vi "Part 1.vi"(7 "Steps":i32=10, 11 "Input":string) -> (3 "Output":i64)   [LabVIEW 2021]
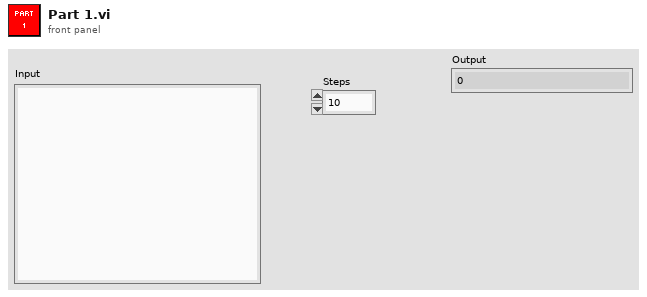
[diagram p1: front panel]
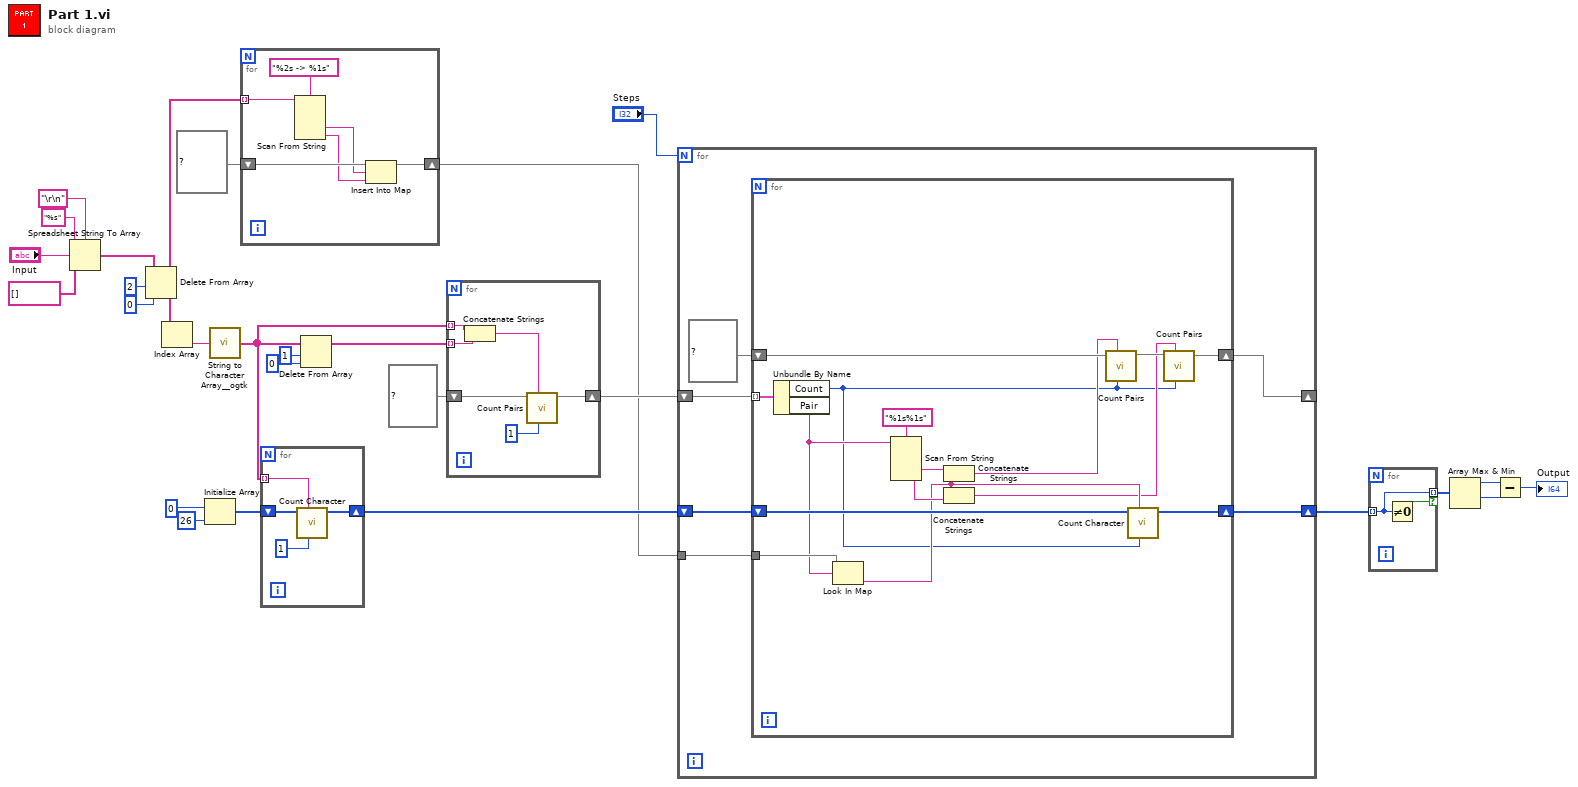
[diagram p0: block diagram]
diagram:
  n1 = Spreadsheet String To Array(delimiter (Tab)="\r\n", format string="%s", spreadsheet string="Input", array type (2D Dbl)=string[] []) -> (array=w24:string[])
  n2 = Delete From Array(array=w24, length=2, index=0) -> (deleted portion=w21:string[], array with subset deleted=w5:string[])
  n3 = Index Array(array=w21) -> (element=w20:string)  [unwired: 1 in]
  n4 = Initialize Array(i64 0, 26 ("dimension size")) -> (w17:i64[])
  n5 = call <userlib>:"String to Character Array__ogtk.vi"("Input String"=w20) -> ("Character Array"=w13:string[])
  n6 = for {
    shift-right: [w34] -> w3
    shift-left: map{string, string} {} ("Pair Map Out") -> [w33]
    tunnel: w5 -> [w32] mode=indexing
    n7 = Scan From String(format string="%2s -> %1s", input string=w32) -> (output 1=w30:string, output 2=w29:string)  [unwired: 4 in, 3 out]
    n8 = Insert Into Map(map in=w33, key=w30, value=w29) -> (map out=w34:map{string, string})  [unwired: 2 out]
  }
  n9 = for {
    tunnel: w13 -> [w37] mode=indexing
    shift-right: [w36] -> w9
    shift-left: w17 -> [w38]
    n10 = call "Count Character.vi"("Amount"=i64 1, "Character"=w37, "Count In"=w38) -> ("Count Out"=w36:i64[])  [unwired: 8 in]
  }
  n11 = Delete From Array(array=w13, length=1, index=0) -> (array with subset deleted=w14:string[])  [unwired: 1 out]
  n12 = for {
    tunnel: w14 -> [w44] mode=indexing
    tunnel: w13 -> [w43] mode=indexing
    shift-right: [w41] -> w10
    shift-left: map{string, i64} {} ("Pair Map Out") -> [w40]
    n13 = Concatenate Strings(w43, w44) -> (w42:string)
    n14 = call "Count Pairs.vi"("Amount"=1, "Pair"=w42, "Pair Map In"=w40) -> ("Pair Map Out"=w41:map{string, i64})  [unwired: 8 in]
  }
  n15 = for {
    N: "Steps" -> [_]
    shift-right: [w48] -> _
    shift-left: w10 -> [w50]
    shift-right: [w46] -> w2
    shift-left: w9 -> [w47]
    tunnel: w3 -> [w45]
    n16 = for {
      tunnel: w50 -> [w64] mode=indexing
      shift-right: [w65] -> w48
      shift-left: map{string, i64} {} ("Pair Map Out") -> [w63]
      shift-right: [w61] -> w46
      shift-left: w47 -> [w62]
      tunnel: w45 -> [w57]
      n17 = Unbundle By Name(w64) -> ("Count"=w51:i64, "Pair"=w56:string)
      n18 = Look In Map(map=w57, key=w56) -> (value=w55:string)  [unwired: 1 in, 1 out]
      n19 = Scan From String(format string="%1s%1s", input string=w56) -> (output 1=w59:string, output 2=w58:string)  [unwired: 4 in, 3 out]
      n20 = Concatenate Strings(w59, w55) -> (w53:string)
      n21 = Concatenate Strings(w55, w58) -> (w52:string)
      n22 = call "Count Pairs.vi"("Amount"=w51, "Pair"=w53, "Pair Map In"=w63) -> ("Pair Map Out"=w54:map{string, i64})  [unwired: 8 in]
      n23 = call "Count Character.vi"("Amount"=w51, "Character"=w55, "Count In"=w62) -> ("Count Out"=w61:i64[])  [unwired: 8 in]
      n24 = call "Count Pairs.vi"("Amount"=w51, "Pair"=w52, "Pair Map In"=w54) -> ("Pair Map Out"=w65:map{string, i64})  [unwired: 8 in]
    }
  }
  n25 = for {
    tunnel: w2 -> [w67] mode=indexing
    tunnel: [w67] -> w1 mode=indexing if=w66
    n26 = Not Equal To 0?(x=w67) -> (x != 0?=w66:bool)
  }
  n27 = Array Max & Min(array=w1) -> (max value=w8:i64, min value=w7:i64)  [unwired: 2 out]
  n28 = Subtract(x=w8, y=w7) -> (x-y=→"Output":i64)
